vi "Laser - Data2Distance (SubVI).vi"(11 "Raw Data":dbl[](array[numeric])) -> (3 "Distance Values":dbl[](array[numeric]))   [LabVIEW 2020]
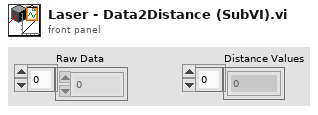
[diagram p1: front panel]
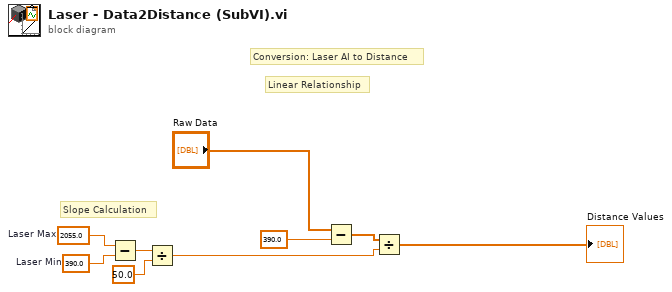
[diagram p0: block diagram]
diagram:
  w1 = 390.0  # Laser Min
  w2 = 2055.0  # Laser Max
  # "Conversion: Laser AI to Distance"
  # "Linear Relationship"
  # "Slope Calculation"
  n1 = Subtract(x=w2, y=w1) -> (x-y=w3:dbl)
  n2 = Divide(x=w3, y=50.0) -> (x/y=w8:dbl)
  n3 = Subtract(x="Raw Data", y=390.0) -> (x-y=w7:dbl[])
  n4 = Divide(x=w7, y=w8) -> (x/y=→"Distance Values":dbl[])
